vi "Env.global.vi"() -> ()   [LabVIEW 2014]
panel:
  in  "Env":variant
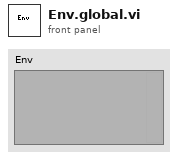
[diagram p1: front panel]
diagram:
